vi "PRIVATE.panel.vi"(0 "object ref":refnum<vi>, 5 "error in (no error)":errorcluster) -> (19 "error out":errorcluster)   [LabVIEW 2012]
doc: "This is just an example for a GUI thread.\n\nLicense Agreement for this software:\n\nCopyright (C)\nGesellschaft für Schwerionenforschung, GSI\nPlanckstr. 1\n64291 Darmstadt\nGermany\n\nContact: D.Beck@gsi.de \n\nThis program is free software; you can redistribute it and/or modify it under the terms of the GNU General Public License as published by the Free Software Foundation; either version 2 of the license, or (at your option) any later version.\n\nThis program is distributed in the hope that it will be useful, but WITHOUT ANYW ARRANTY; without even the implied warranty of MERCHANTABILITY or FITNESS FOR A PARTICULAR PURPOSE. See the GNU General License for more details (http://www.gnu.org).\n\nGesellschaft für Schwerionenforschung, GSI\nPlanckstr. 1, 64291 Darmstadt, Germany\nFor all questions and ideas contact: M.Richter@gsi.de, H.Brand@gsi.de or D.Beck@gsi.de.\nLast update: 18-DEC-2002"
uses:
  CSCore/CSSystem/CSSystemLib/CSSystemLib.lvlib
panel:
  in  "stop":bool
  out "loop counter":i32
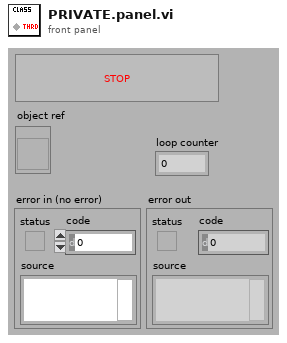
[diagram p1: front panel]
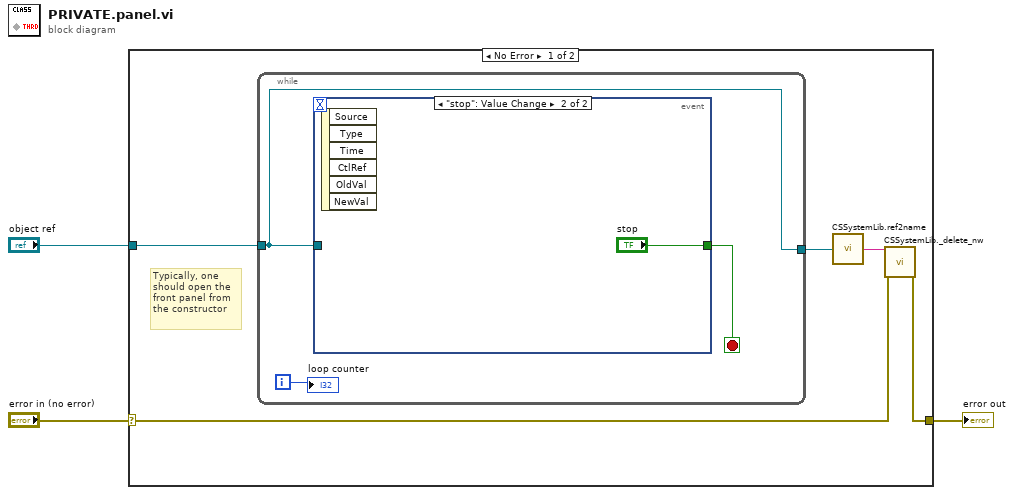
[diagram p0: block diagram]
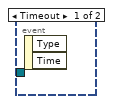
[diagram p2: hidden frame]
diagram:
  n1 = case shown="No Error" "error in (no error)" {
    selector: "error in (no error)" -> [w4 w13]
    tunnel: [w8 w13] -> w2
    tunnel: "object ref" -> [w7 _]
    frame No Error {
      # "Typically, one\nshould open the\nfront panel from\nthe constructor"
      n2 = while {
        tunnel: w7 -> [w9]
        tunnel: [w9] -> w6
        i -> [w10]
        stop <- w11 stop-if-true
        n3 = event shown="[1] \"stop\": Value Change" {
          selector: _ -> [_ _]
          dyn-events: _ -> [_ _]
          timeout: _ -> [_ _]
          tunnel: [_ "stop"] -> w11
          tunnel: w9 -> [_ _]
          event Timeout {
            n4 = event-data() -> ()  [unwired: 1 in, 2 out]
          }
          event "stop": Value Change {
            n5 = event-data() -> ()  [unwired: 1 in, 6 out]
          }
        }
        "loop counter" <- w10
      }
      n6 = call "CSSystemLib.ref2name.vi"("obj refnum"=w6) -> ("name"=w5:string)
      n7 = call "CSSystemLib._delete_nw.vi"("objectName"=w5, "error in (no error)"=w4) -> ("error out"=w8:errorcluster)  [unwired: 17 in]
    }
    frame Error {
    }
  }
  "error out" <- w2
